vi "Queue.vi"(6 "AtOpposite":bool, 7 "Function":T1(ring), 8 "error in (no error)":errorcluster, 9 "DataIN":variant[](array[variant]), 10 "ActionsIN":string[](array[string]), 11 "QueueName":string) -> (0 "error out":errorcluster, 1 "DataOut":variant, 2 "ActionsOut":string)   [LabVIEW 2018]
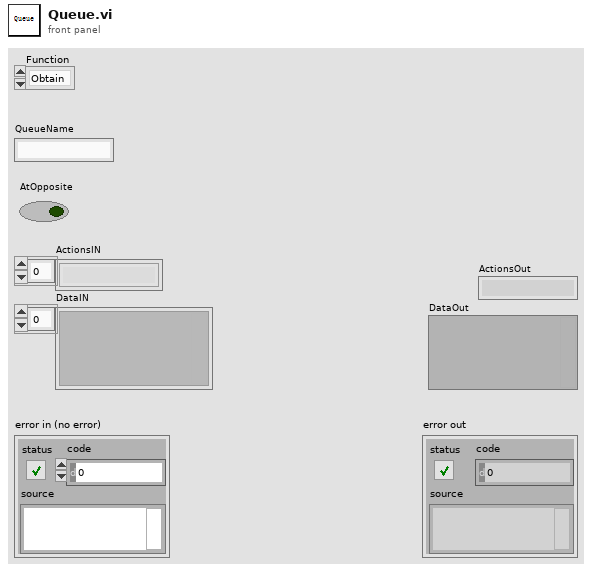
[diagram p1: front panel]
types:
  T1 = enum16{"Obtain", "Enqueue", "Dequeue", "Release"}
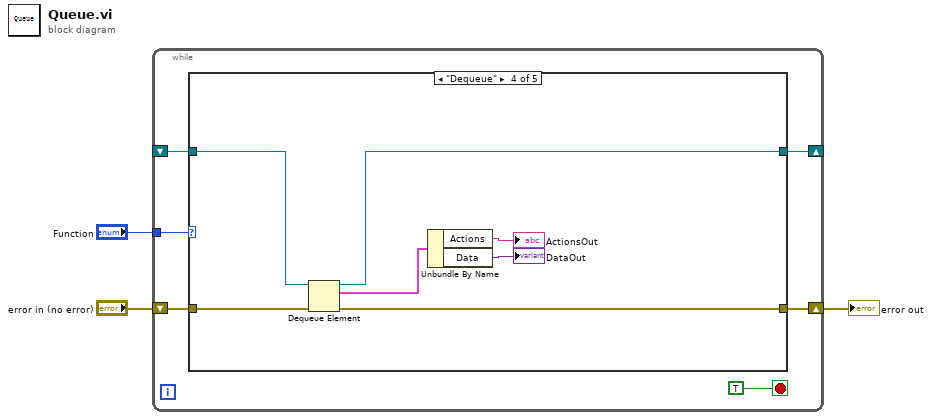
[diagram p0: block diagram]
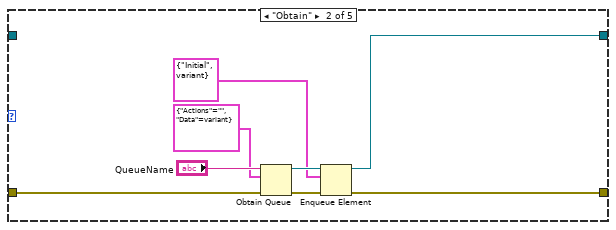
[diagram p3: hidden frame]
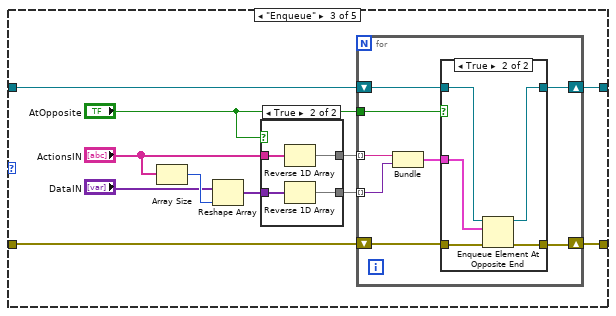
[diagram p4: hidden frame]
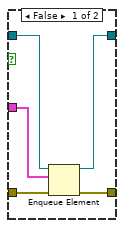
[diagram p6: hidden frame]
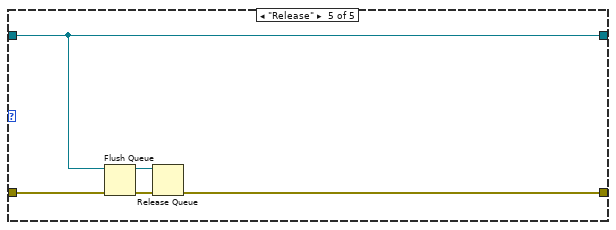
[diagram p7: hidden frame]
diagram:
  n1 = while {
    tunnel: "Function" -> [w8]
    shift-right: [w5] -> _
    shift-left: _ -> [w4]
    shift-right: [w6] -> w1
    shift-left: "error in (no error)" -> [w7]
    stop <- TRUE stop-if-true
    n2 = case shown="\"Dequeue\"" w8 {
      tunnel: w7 -> [w10 w17 w22 w58 w64]
      tunnel: [w10 w13 w23 w55 w63] -> w6
      tunnel: [w11 w12 w21 w56 w62] -> w5
      tunnel: w4 -> [w11 _ w20 w57 w62]
      frame Default {
      }
      frame "Obtain" {
        n3 = Obtain Queue(name (unnamed)="QueueName", element data type=cluster{"Actions":string, "Data":variant} {"Actions"="", "Data"=variant}, error in (no error)=w17) -> (queue out=w18:refnum<queue>, error out=w14:errorcluster)  [unwired: 2 in, 1 out]
        n4 = Enqueue Element(queue=w18, element=cluster{"Actions":string, "Data":variant} {"Actions"="Initial", "Data"=variant} ("元素"), error in (no error)=w14) -> (queue out=w12:refnum<queue>, error out=w13:errorcluster)  [unwired: 2 out]
      }
      frame "Enqueue" {
        n5 = Array Size(array="ActionsIN") -> (size(s)=w27:i32)
        n6 = Reshape Array("DataIN", w27) -> (w26:variant[])
        n7 = case shown="True" "AtOpposite" {
          tunnel: "ActionsIN" -> [w32 w36]
          tunnel: w26 -> [w31 w35]
          tunnel: [w32 w34] -> w29
          tunnel: [w31 w33] -> w30
          frame False {
          }
          frame True {
            n8 = Reverse 1D Array(array=w36) -> (reversed array=w34:string[])
            n9 = Reverse 1D Array(array=w35) -> (reversed array=w33:variant[])
          }
        }
        n10 = for {
          tunnel: "AtOpposite" -> [w44]
          tunnel: w29 -> [w41] mode=indexing
          tunnel: w30 -> [w40] mode=indexing
          shift-right: [w37] -> w23
          shift-left: w22 -> [w42]
          shift-right: [w38] -> w21
          shift-left: w20 -> [w43]
          n11 = Bundle("字符串"=w41, "变体"=w40) -> (w39:cluster{"字符串":string, "变体":variant})  [unwired: 1 out]
          n12 = case shown="True" w44 {
            tunnel: w43 -> [w48 w54]
            tunnel: w42 -> [w45 w50]
            tunnel: w39 -> [w49 w53]
            tunnel: [w47 w52] -> w38
            tunnel: [w46 w51] -> w37
            frame False {
              n13 = Enqueue Element(queue=w48, element=w49, error in (no error)=w45) -> (queue out=w47:refnum<queue>, error out=w46:errorcluster)  [unwired: 2 out]
            }
            frame True {
              n14 = Enqueue Element At Opposite End(queue=w54, element=w53, error in (no error)=w50) -> (queue out=w52:refnum<queue>, error out=w51:errorcluster)  [unwired: 2 out]
            }
          }
        }
      }
      frame "Dequeue" {
        n15 = Dequeue Element(queue=w57, error in (no error)=w58) -> (queue out=w56:refnum<queue>, element=w61:cluster{"Actions":string, "Data":variant}, error out=w55:errorcluster)  [unwired: 2 out]
        n16 = Unbundle By Name(w61) -> ("Actions"=→"ActionsOut":string, "Data"=→"DataOut":variant)
      }
      frame "Release" {
        n17 = Flush Queue(queue=w62, error in (no error)=w64) -> (queue out=w66:refnum<queue>, error out=w65:errorcluster)  [unwired: 1 out]
        n18 = Release Queue(queue=w66, error in (no error)=w65) -> (error out=w63:errorcluster)  [unwired: 3 out]
      }
    }
  }
  "error out" <- w1
